vi "setIVmode.vi"(8 "error in (no error)":errorcluster, 10 "IV mode":bool) -> (0 "error out":errorcluster)   [LabVIEW 2016]
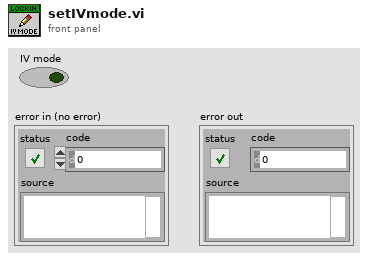
[diagram p1: front panel]
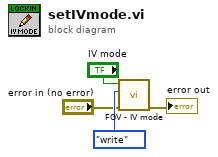
[diagram p0: block diagram]
diagram:
  n1 = call "FGV - IV mode.vi"("error in"="error in (no error)", "Function"=enum16{"write", "read"}."write", "IV mode"="IV mode") -> ("error out"=→"error out":errorcluster)  [unwired: 3 in, 1 out]
